vi "Set_Parameter_Instrument (Json).vi"(8 "error in (no error)":errorcluster caption="entrée d'erreur (pas d'erreur)", 10 "Parameter (Json)":string, 11 "Show_Information en entrée":refnum<class "Remove_Weight.lvclass">) -> (0 "error out":errorcluster caption="sortie d'erreur", 3 "Show_Information en sortie":refnum<class "Remove_Weight.lvclass">)   [LabVIEW 2020, in "Library Test.lvlib" / "Remove_Weight.lvclass"]
uses:
  Remove_Weight.lvclass
  C:/Users/ngarcin/OneDrive - Altyor/Standard TB/Class/Test/Test (Default)/Test (Default).lvclass
  Remove_Weight.lvclass/Remove_Weight.ctl
  JSON API/JSON Value/Set from JSON string.vi
  Test_Without_Instr/Test_Without_Inst.lvclass
  Instrument/Instrument (Default)/Class Instrument (Default).lvclass
  JSON API/JSON Value/JSON Value.lvclass
  JSON API/Variant JSON/Variant JSON.lvlib
  JSON API/Get Polymorphic/JSON GetSet.lvlib
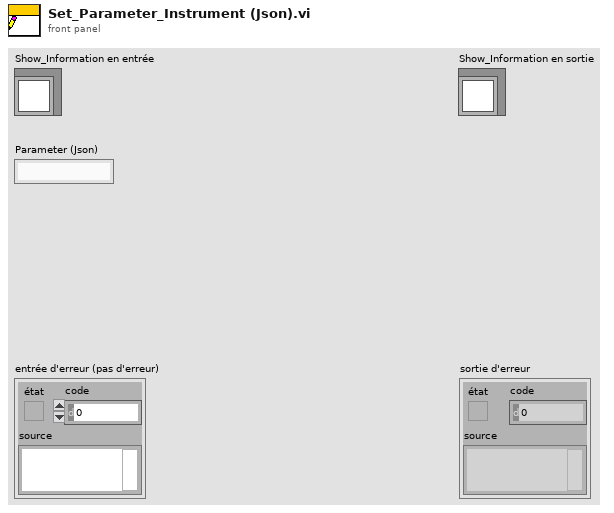
[diagram p1: front panel]
types:
  T1 = cluster{"Information_Operator":string, "Path_Picture":path, "Timeout (ms)":u64, "Weight":dbl}
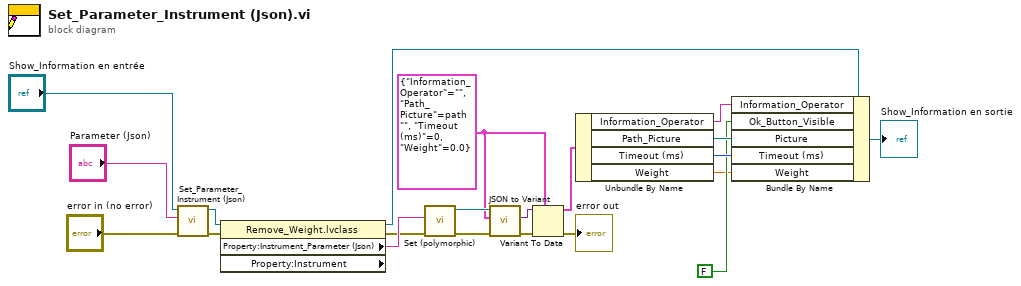
[diagram p0: block diagram]
diagram:
  w5 = T1 {"Information_Operator"="", "Path_Picture"=path "", "Timeout (ms)"=0, "Weight"=0.0} ("Cluster des données privées de classe")
  n1 = call-parent "Set_Parameter_Instrument (Json).vi"("error in (no error)"="error in (no error)", "Parameter (Json)"="Parameter (Json)", "Test (Default) en entrée"="Show_Information en entrée") -> ("error out"=w11:errorcluster, "Test (Default) en sortie"=w12:refnum<class "Remove_Weight.lvclass">)  [unwired: 7 in]
  n2 = property class="Remove_Weight.lvclass" props=["Property:Instrument_Parameter (Json)", "Property:Instrument"](reference=w12, error in=w11) -> (reference out=w10:refnum<class "Remove_Weight.lvclass">, error out=w17:errorcluster, "Property:Instrument_Parameter (Json)"=w18:string)  [unwired: 1 out]
  n3 = call-poly "Set (polymorphic).vi"("error in (no error)"=w17, "JSON stream"=w18) -> ("error out"=w14:errorcluster, "JSON Value out"=w16:refnum<class "JSON Value.lvclass">)  [unwired: 7 in, 1 out]
  n4 = call "JSON to Variant.vi"("error in (no error)"=w14, "Variant (Data Type)"=w5, "JSON Value"=w16) -> ("error out"=w15:errorcluster, "Variant out"=w13:variant)  [unwired: 7 in]
  n5 = Variant To Data(error in=w15, type=w5, Variant=w13) -> (data=w9:T1, error out=→"error out":errorcluster)
  n6 = Unbundle By Name(w9) -> ("Information_Operator"=w8:string, "Path_Picture"=w7:path, "Timeout (ms)"=w6:u64, "Weight"=w1:dbl)
  n7 = Bundle By Name(cluster=w10, "Information_Operator"=w8, "Ok_Button_Visible"=FALSE, "Picture"=w7, "Timeout (ms)"=w6, "Weight"=w1) -> (→"Show_Information en sortie":refnum<class "Remove_Weight.lvclass">)
